vi "Main.vi"() -> ()   [LabVIEW 2009]
doc: "黑白棋\n如果您想使用此程序请与作者联系。\n作者：genreeze\n联系方式：genreeze@126.com"
uses:
  Controls/Chess.ctl
  Controls/States.ctl
  Controls/StateEvents.ctl
  Classes/Player/Player.lvclass
  Controls/directions.ctl
panel:
  in  "终局":bool
  out "Tab Control":enum32{"Page 1", "Page 2"}(tab)
  in  "Chesspiece 2":u16(ring)=1
  in  "Chesspiece":u16(ring)=1
  in  "Start":bool
  in  "Exit":bool
  in  "StateEvent":T1
  in  "States":T2
  out "Chessboard":T3
  # "黑方"
  # "白方"
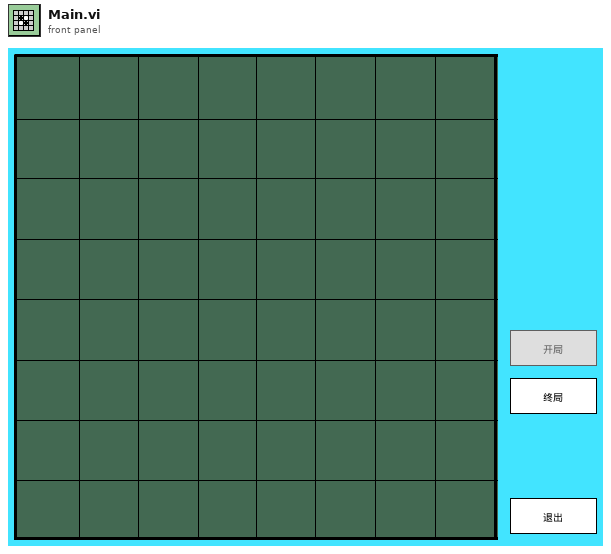
[diagram p1: front panel]
types:
  T1 = typedef "StateEvents.ctl" = cluster{"Initialize":refnum<user-event>, "ShiftPlayer":refnum<user-event>, "TurnOver":refnum<user-event>, "Auto":refnum<user-event>, "JudgeResult":refnum<user-event>, "Wait":refnum<user-event>, "ShowResult":refnum<user-event>, "Idle":refnum<user-event>}
  T2 = typedef "States.ctl" = cluster{"Initialize":string, "ShiftPlayer":string, "TurnOver":string, "Auto":string, "JugeResult":string, "Wait":string, "ShowResult":string, "Idle":string}
  T3 = typedef "Chess.ctl" = u16[][]
  T4 = enum8{"Enabled", "Disabled", "Disabled and Grayed Out"}
  T5 = typedef "directions.ctl" = enum16{"Left", "Right", "Top", "Bottom", "TopLeft", "TopRight", "BottomLeft", "BottomRight", "ClearAll", "ReadAll"}
  T6 = typedef "ItemIndex.ctl" = cluster{"Row":i32, "Col":i32}
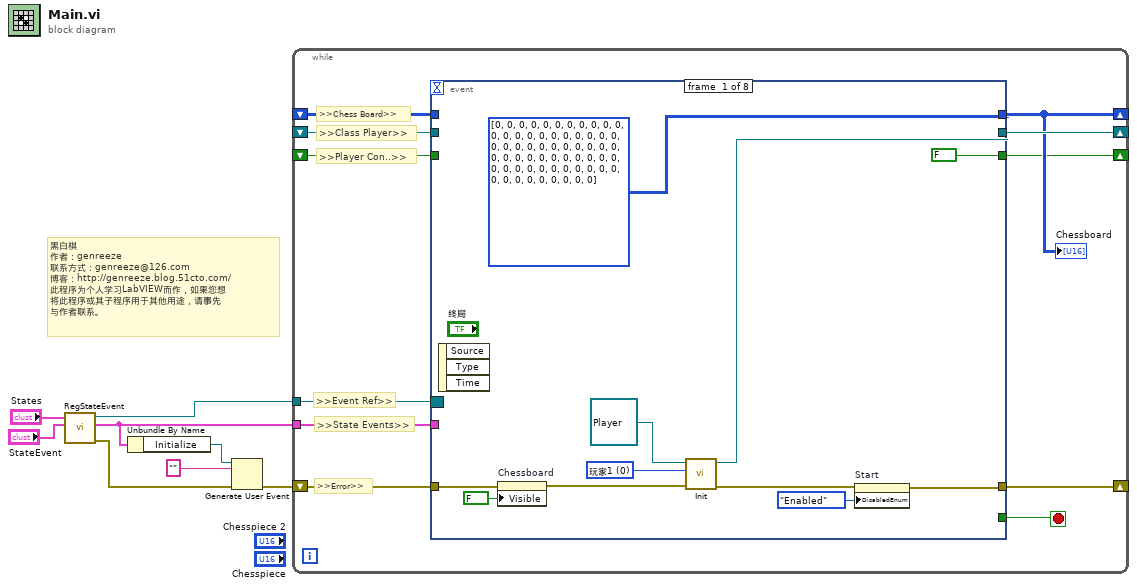
[diagram p0: block diagram]
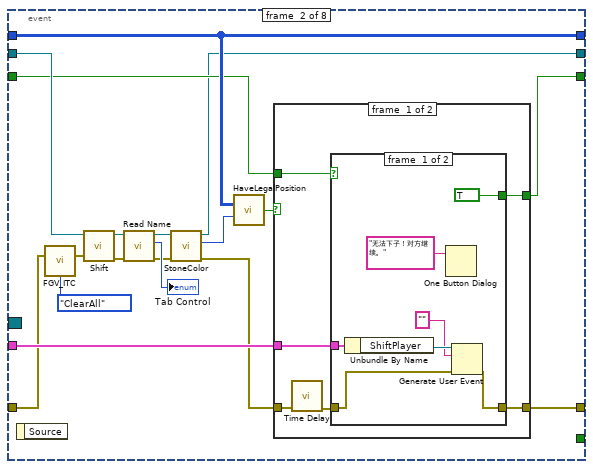
[diagram p2: hidden frame]
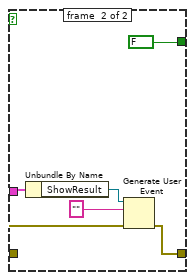
[diagram p3: hidden frame]
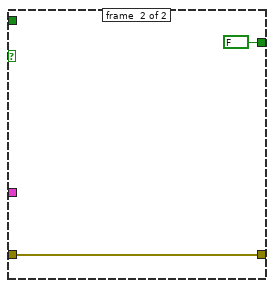
[diagram p4: hidden frame]
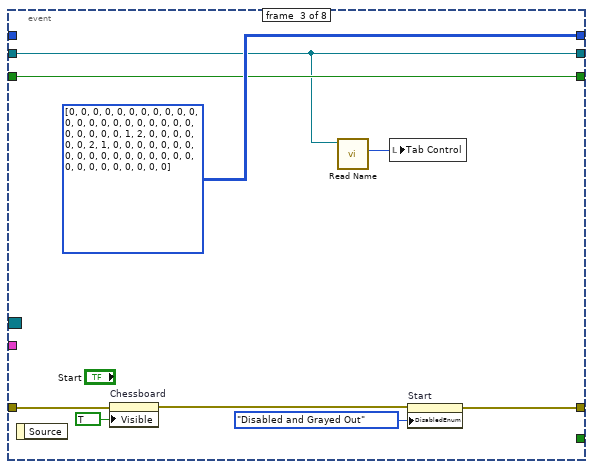
[diagram p5: hidden frame]
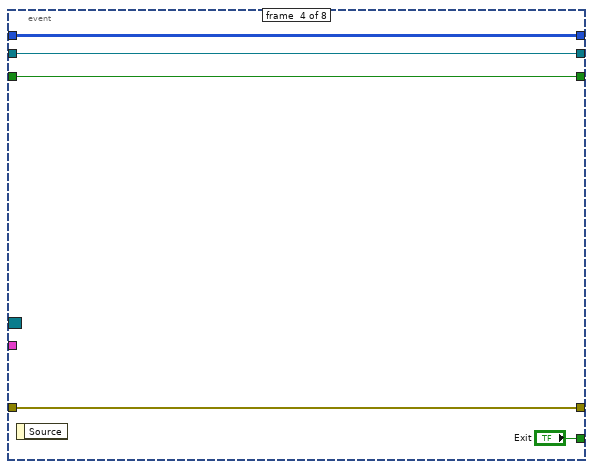
[diagram p6: hidden frame]
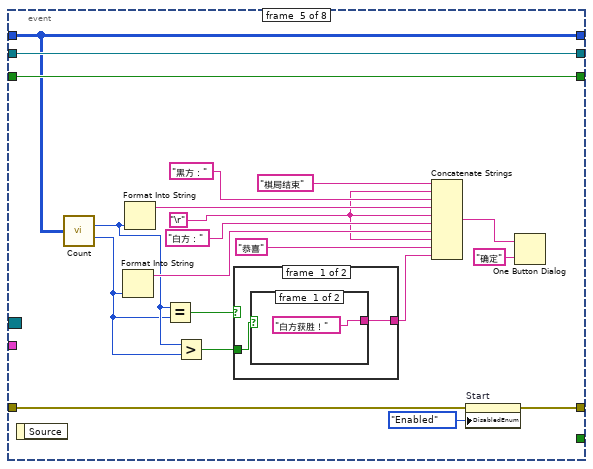
[diagram p7: hidden frame]
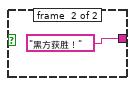
[diagram p8: hidden frame]
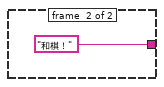
[diagram p9: hidden frame]
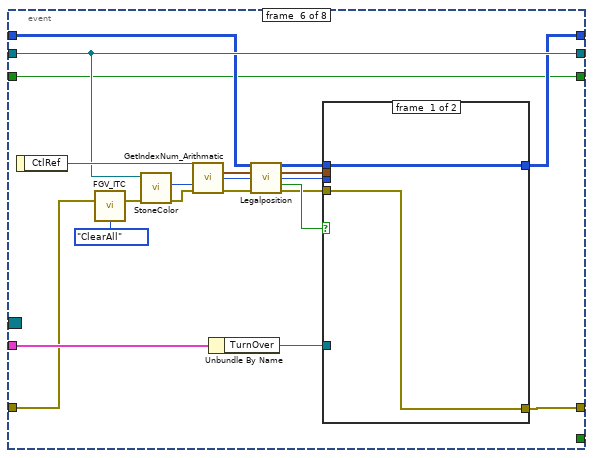
[diagram p10: hidden frame]
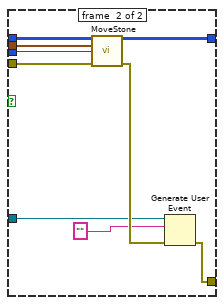
[diagram p11: hidden frame]
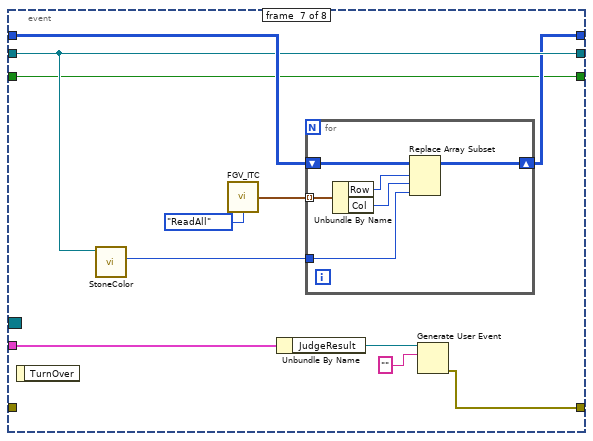
[diagram p12: hidden frame]
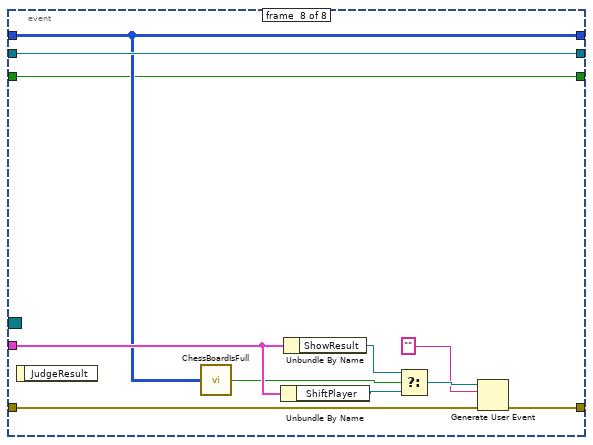
[diagram p13: hidden frame]
diagram:
  # "黑白棋\n作者：genreeze\n联系方式：genreeze@126.com\n博客：http://genreeze.blog.51cto.com/\n此程序为个人学习LabVIEW而作，如果您想\n将此程序或其子程序用于其他用途，请事先\n与作者联系。"
  n1 = call "RegStateEvent.vi"("StateEvent"="StateEvent", "States"="States") -> ("error out"=w5:errorcluster, "StateEvent(out)"=w3:T1, "Event Registration Refnum"=w1:refnum<event-registration>)  [unwired: 7 in]
  n2 = Unbundle By Name(w3) -> ("Initialize"=w4:refnum<user-event>)
  n3 = Generate User Event(user event=w4, event data cluster="" ("event data"), error in=w5) -> (error out=w2:errorcluster)  [unwired: 1 out]
  n4 = while {
    tunnel: w3 -> [w19]
    tunnel: w1 -> [w11]
    shift-right: [w17] -> _
    shift-left: w2 -> [w18]
    shift-right: [w12] -> _
    shift-left: _ -> [w13]
    shift-right: [w15] -> _
    shift-left: _ -> [w16]
    shift-right: [w10] -> _
    shift-left: _ -> [w9]
    stop <- w14 stop-if-true
    # ">>Player Con..>>"
    # ">>Class Player>>"
    # ">>Chess Board>>"
    # ">>Event Ref>>"
    # ">>State Events>>"
    # ">>Error>>"
    n5 = event shown="[1] <StateEvent.ShiftPlayer>: User Event" {
      selector: w11 -> [_ _ _ _ _ _ _ _]
      dyn-events: _ -> [_ _ _ _ _ _ _ _]
      timeout: _ -> [_ _ _ _ _ _ _ _]
      tunnel: w19 -> [_ w44 _ _ _ w128 w144 w166]
      tunnel: w18 -> [w24 w38 w76 w80 w99 w111 _ w161]
      tunnel: [w22 w46 w70 w80 w100 w113 w141 w160] -> w17
      tunnel: [T3 [[0, 0, 0, 0, 0, 0, 0, 0], [0, 0, 0, 0, 0, 0, 0, 0], [0, 0, 0, 0, 0, 0, 0, 0], [0, 0, 0, 0, 0, 0, 0, 0], [0, 0, 0, 0, 0, 0, 0, 0], [0, 0, 0, 0, 0, 0, 0, 0], [0, 0, 0, 0, 0, 0, 0, 0], [0, 0, 0, 0, 0, 0, 0, 0]] ("Chessboard") w48 T3 [[0, 0, 0, 0, 0, 0, 0, 0], [0, 0, 0, 0, 0, 0, 0, 0], [0, 0, 0, 0, 0, 0, 0, 0], [0, 0, 0, 1, 2, 0, 0, 0], [0, 0, 0, 2, 1, 0, 0, 0], [0, 0, 0, 0, 0, 0, 0, 0], [0, 0, 0, 0, 0, 0, 0, 0], [0, 0, 0, 0, 0, 0, 0, 0]] ("Chessboard") w83 w101 w115 w145 w158] -> w12
      tunnel: w13 -> [_ w48 _ w83 w101 w124 w148 w158]
      tunnel: w16 -> [_ w45 w74 w81 w103 w125 w147 w167]
      tunnel: [w28 w31 w74 w81 w103 w125 w147 w167] -> w15
      tunnel: [_ _ _ "Exit" _ _ _ _] -> w14
      tunnel: [FALSE w42 w75 w79 w102 w112 w140 w157] -> w10
      tunnel: w9 -> [_ w43 w75 w79 w102 w112 w140 w157]
      event #0 {
        w29 = u16 0 items=["玩家1", "玩家2"] ("Name")
        n6 = event-data() -> ()  [unwired: 1 in, 3 out]
        n7 = property on="Chessboard" class="Arr (strict)"(error in=w24, "Visible"=FALSE) -> (error out=w23:errorcluster)  [unwired: 1 in, 1 out]
        n8 = call "Init.vi"("error in (no error)"=w23, "Name"=w29, "Player in"=refnum<class "Player.lvclass"> refnum ("Player.lvclass")) -> ("error out"=w21:errorcluster, "Player out"=w28:refnum<class "Player.lvclass">)  [unwired: 7 in]
        n9 = property on="Start" class="Bool"(error in=w21, "DisabledEnum"=T4."Enabled" ("Disabled")) -> (error out=w22:errorcluster)  [unwired: 1 in, 1 out]
      }
      event #1 {
        n10 = event-data() -> ()  [unwired: 1 in, 1 out]
        n11 = call "FGV_ITC.vi"("error in (no error)"=w38, "Action"=directions."ClearAll") -> ("error out"=w37:errorcluster)  [unwired: 12 in, 1 out]
        n12 = call "Shift.vi"("error in (no error)"=w37, "Player in"=w45) -> ("error out"=w36:errorcluster, "Player out"=w35:refnum<class "Player.lvclass">)  [unwired: 8 in]
        n13 = call "Read Name.vi"("error in (no error)"=w36, "Player in"=w35) -> ("error out"=w33:errorcluster, "Name"=→"Tab Control":u16, "Player out"=w34:refnum<class "Player.lvclass">)  [unwired: 7 in]
        n14 = call "StoneColor.vi"("error in (no error)"=w33, "Player in"=w34) -> ("error out"=w32:errorcluster, "StoneColor"=w41:u16, "Player out"=w31:refnum<class "Player.lvclass">)  [unwired: 7 in]
        n15 = call "HaveLegalPosition.vi"("ChessBoard"=w48, "StoneColor"=w41) -> ("HaveLegalPlace?"=w47:bool)  [unwired: 13 in]
        n16 = case shown="False" w47 {
          tunnel: w44 -> [w52 _]
          tunnel: w32 -> [w50 w69]
          tunnel: [w51 w69] -> w46
          tunnel: w43 -> [w54 _]
          tunnel: [w53 FALSE] -> w42
          frame #0 {
            n17 = call "Time Delay"("error in (no error)"=w50) -> ("error out"=w49:errorcluster)  [unwired: 10 in]
            n18 = case shown="False" w54 {
              tunnel: [TRUE FALSE] -> w53
              tunnel: w52 -> [w59 w66]
              tunnel: w49 -> [w56 w64]
              tunnel: [w55 w63] -> w51
              frame #0 {
                n19 = Unbundle By Name(w59) -> ("ShiftPlayer"=w58:refnum<user-event>)
                n20 = One Button Dialog(message="无法下子！对方继续。") -> ()  [unwired: 1 in, 1 out]
                n21 = Generate User Event(user event=w58, event data cluster="" ("event data"), error in=w56) -> (error out=w55:errorcluster)  [unwired: 1 out]
              }
              frame #1 {
                n22 = Unbundle By Name(w66) -> ("ShowResult"=w65:refnum<user-event>)
                n23 = Generate User Event(user event=w65, event data cluster="" ("event data"), error in=w64) -> (error out=w63:errorcluster)  [unwired: 1 out]
              }
            }
          }
          frame #1 {
          }
        }
      }
      event #2 {
        n24 = event-data() -> ()  [unwired: 1 in, 1 out]
        n25 = property on="Chessboard" class="Arr (strict)"(error in=w76, "Visible"=TRUE) -> (error out=w71:errorcluster)  [unwired: 1 in, 1 out]
        n26 = call "Read Name.vi"("Player in"=w74) -> ("Name"=w73:u16)  [unwired: 8 in, 2 out]
        n27 = local write "Tab Control"(w73) -> ()
        n28 = property on="Start" class="Bool"(error in=w71, "DisabledEnum"=T4."Disabled and Grayed Out" ("Disabled")) -> (error out=w70:errorcluster)  [unwired: 1 in, 1 out]
      }
      event #3 {
        n29 = event-data() -> ()  [unwired: 1 in, 1 out]
      }
      event #4 {
        w85 = "\r"
        n30 = event-data() -> ()  [unwired: 1 in, 1 out]
        n31 = call "Count.vi"("Chess board"=w101) -> ("BlackNum"=w89:u16, "WhiteNum"=w88:u16)  [unwired: 13 in]
        n32 = Format Into String(w88) -> (resulting string=w93:string)  [unwired: 3 in, 1 out]
        n33 = Format Into String(w89) -> (resulting string=w95:string)  [unwired: 3 in, 1 out]
        n34 = Equal?(x=w89, y=w88) -> (x = y?=w90:bool)
        n35 = Greater?(x=w89, y=w88) -> (0:w87:bool)
        n36 = case shown="False" w90 {
          tunnel: w87 -> [w105 _]
          tunnel: [w104 "和棋！" ("string")] -> w86
          frame #0 {
            n37 = case shown="False" w105 {
              tunnel: ["白方获胜！" ("string") "黑方获胜！" ("string")] -> w104
              frame #0 {
              }
              frame #1 {
              }
            }
          }
          frame #1 {
          }
        }
        n38 = Concatenate Strings("棋局结束" ("string"), w85, "黑方：" ("button name (\"OK\")"), w95, w85, "白方：" ("string"), w93, w85, "恭喜" ("string"), w86) -> (w92:string)
        n39 = property on="Start" class="Bool"(error in=w99, "DisabledEnum"=T4."Enabled" ("Disabled")) -> (error out=w100:errorcluster)  [unwired: 1 in, 1 out]
        n40 = One Button Dialog(message=w92, button name ("OK")="确定") -> ()  [unwired: 1 out]
      }
      event #5 {
        n41 = event-data() -> ("CtlRef"=w127:refnum<vi>)  [unwired: 1 in]
        n42 = call "FGV_ITC.vi"("error in (no error)"=w111, "Action"=directions."ClearAll") -> ("error out"=w110:errorcluster)  [unwired: 12 in, 1 out]
        n43 = call "StoneColor.vi"("error in (no error)"=w110, "Player in"=w125) -> ("error out"=w126:errorcluster, "StoneColor"=w121:u16)  [unwired: 7 in, 1 out]
        n44 = call "GetIndexNum_Arithmatic.vi"("ArrayRef"=w127, "error in (no error)"=w126) -> ("ItemIndex"=w123:T6, "error out"=w122:errorcluster)  [unwired: 11 in, 1 out]
        n45 = Unbundle By Name(w128) -> ("TurnOver"=w114:refnum<user-event>)
        n46 = call "Legalposition.vi"("Chessboard"=w124, "ItemIndex"=w123, "StoneColor"=w121, "error in (no error)"=w122) -> ("Chessboard out"=w117:T3, "ItemIndex out"=w116:T6, "StoneColor out"=w118:u16, "Legal?"=w120:bool, "error out"=w119:errorcluster)  [unwired: 7 in]
        n47 = case shown="True" w120 {
          tunnel: [w130 w138] -> w113
          tunnel: [w129 w139] -> w115
          tunnel: w119 -> [w130 w135]
          tunnel: w118 -> [_ w134]
          tunnel: w117 -> [w129 w133]
          tunnel: w116 -> [_ w132]
          tunnel: w114 -> [_ w131]
          frame #0 {
          }
          frame #1 {
            n48 = call "MoveStone.vi"("Chessboard"=w133, "ItemIndex"=w132, "StoneColor"=w134, "error in (no error)"=w135) -> ("output array"=w139:T3, "error out"=w137:errorcluster)  [unwired: 9 in, 1 out]
            n49 = Generate User Event(user event=w131, event data cluster="" ("event data"), error in=w137) -> (error out=w138:errorcluster)  [unwired: 1 out]
          }
        }
      }
      event #6 {
        n50 = event-data() -> ()  [unwired: 1 in, 1 out]
        n51 = call "StoneColor.vi"("Player in"=w147) -> ("StoneColor"=w146:u16)  [unwired: 8 in, 2 out]
        n52 = call "FGV_ITC.vi"("Action"=directions."ReadAll") -> ("ItemsToChange"=w149:T6[])  [unwired: 13 in, 1 out]
        n53 = Unbundle By Name(w144) -> ("JudgeResult"=w143:refnum<user-event>)
        n54 = for {
          tunnel: w149 -> [w155] mode=indexing
          tunnel: w146 -> [w152]
          shift-right: [w151] -> w145
          shift-left: w148 -> [w156]
          n55 = Unbundle By Name(w155) -> ("Row"=w154:i32, "Col"=w153:i32)
          n56 = Replace Array Subset(array=w156, new element=w152, index (row)=w154, index (col)=w153) -> (w151:T3)
        }
        n57 = Generate User Event(user event=w143, event data cluster="" ("event data")) -> (error out=w141:errorcluster)  [unwired: 1 in, 1 out]
      }
      event #7 {
        n58 = event-data() -> ()  [unwired: 1 in, 1 out]
        n59 = call "ChessBoardIsFull.vi"("ChessBoard"=w158) -> ("Full?"=w159:bool)  [unwired: 14 in]
        n60 = Unbundle By Name(w166) -> ("ShiftPlayer"=w164:refnum<user-event>)
        n61 = Unbundle By Name(w166) -> ("ShowResult"=w165:refnum<user-event>)
        n62 = Select(t=w165, s=w159, f=w164) -> (s? t:f=w163:refnum<user-event>)
        n63 = Generate User Event(user event=w163, event data cluster="" ("event data"), error in=w161) -> (error out=w160:errorcluster)  [unwired: 1 out]
      }
    }
    "Chessboard" <- w12
  }
